vi "nanocal -- nuclear schottky fit -- 2x2 -- V9.vi"() -> ()   [LabVIEW 2021] (continued)
 -> 2.000000000000   ,  \"θ\" -> 45.000000000000   ,  \"Reoff\" -> -2979591.836734697220   ,  \"Imoff\" -> 0.000000000000   ,  \"στ1\" -> 0.135403699680   ,  \"στS\" -> 0.000163058440   ,  \"στN\" -> 0.001967445367    |>   , \n\"IDS0550_220606_RAW_cal__ref_\" ->   <|    \"ζ\" -> 0.030650031864   ,  \"τ1\" -> 0.371061825507   ,  \"τS\" -> 0.019434774268   ,  \"τN\" -> 0.003191687976   ,  \"τC\" -> 0.001854354331   ,  \"κ0\" -> 0.000000005040   ,  \"mm1\" -> 0.000050590010   ,  \"mm2\" -> 0.021630629169   ,  \"mm3\" -> 0.374554924692   ,  \"T\" -> 0.820000000000   ,  \"B\" -> 2.000000000000   ,  \"θ\" -> 45.000000000000   ,  \"Reoff\" -> -1632653.061224489940   ,  \"Imoff\" -> 0.000000000000   ,  \"στ1\" -> 0.107047861270   ,  \"στS\" -> 0.000201030582   ,  \"στN\" -> 0.000503414357    |>   , \n\"IDS0550_220606_RAW_cal__sam_\" ->   <|    \"ζ\" -> 0.000000000000   ,  \"τ1\" -> 0.000000000000   ,  \"τS\" -> 0.000000000000   ,  \"τN\" -> 0.000000000000   ,  \"τC\" -> 0.000000000000   ,  \"κ0\" -> 0.000000000000   ,  \"mm1\" -> 0.000000000000   ,  \"mm2\" -> 0.000000000000   ,  \"mm3\" -> 0.000000000000   ,  \"T\" -> 0.820000000000   ,  \"B\" -> 2.000000000000   ,  \"θ\" -> 45.000000000000   ,  \"Reoff\" -> 0.000000000000   ,  \"Imoff\" -> 0.000000000000   ,  \"στ1\" -> 0.000000000000   ,  \"στS\" -> 0.000000000000   ,  \"στN\" -> 0.000000000000    |>   , \n\"IDS0551_220606_RAW_cal__ref_\" ->   <|    \"ζ\" -> 0.023490949621   ,  \"τ1\" -> 0.378878569703   ,  \"τS\" -> 0.026968462806   ,  \"τN\" -> 0.001819085143   ,  \"τC\" -> 0.002360831644   ,  \"κ0\" -> 0.000000007142   ,  \"mm1\" -> 0.000049999340   ,  \"mm2\" -> 0.029754158704   ,  \"mm3\" -> 0.380899038091   ,  \"T\" -> 1.120000000000   ,  \"B\" -> 2.000000000000   ,  \"θ\" -> 45.000000000000   ,  \"Reoff\" -> -959183.673469387924   ,  \"Imoff\" -> 0.000000000000   ,  \"στ1\" -> 0.190596529331   ,  \"στS\" -> 0.000292683710   ,  \"στN\" -> 0.000959345989    |>   , \n\"IDS0551_220606_RAW_cal__sam_\" ->   <|    \"ζ\" -> 0.000000000000   ,  \"τ1\" -> 0.000000000000   ,  \"τS\" -> 0.000000000000   ,  \"τN\" -> 0.000000000000   ,  \"τC\" -> 0.000000000000   ,  \"κ0\" -> 0.000000000000   ,  \"mm1\" -> 0.000000000000   ,  \"mm2\" -> 0.000000000000   ,  \"mm3\" -> 0.000000000000   ,  \"T\" -> 1.120000000000   ,  \"B\" -> 2.000000000000   ,  \"θ\" -> 45.000000000000   ,  \"Reoff\" -> 0.000000000000   ,  \"Imoff\" -> 0.000000000000   ,  \"στ1\" -> 0.000000000000   ,  \"στS\" -> 0.000000000000   ,  \"στN\" -> 0.000000000000    |>   , \n\"IDS0552_220606_RAW_cal__ref_\" ->   <|    \"ζ\" -> 0.016903896176   ,  \"τ1\" -> 0.389208085767   ,  \"τS\" -> 0.042839293805   ,  \"τN\" -> 0.001054381509   ,  \"τC\" -> 0.002700942117   ,  \"κ0\" -> 0.000000012752   ,  \"mm1\" -> 0.000042315056   ,  \"mm2\" -> 0.046078096141   ,  \"mm3\" -> 0.390424266131   ,  \"T\" -> 1.900000000000   ,  \"B\" -> 2.000000000000   ,  \"θ\" -> 45.000000000000   ,  \"Reoff\" -> -285714.285714285448   ,  \"Imoff\" -> 0.000000000000   ,  \"στ1\" -> 0.071680793743   ,  \"στS\" -> 0.000751471945   ,  \"στN\" -> 0.000020808748    |>   , \n\"IDS0552_220606_RAW_cal__sam_\" ->   <|    \"ζ\" -> 0.000000000000   ,  \"τ1\" -> 0.000000000000   ,  \"τS\" -> 0.000000000000   ,  \"τN\" -> 0.000000000000   ,  \"τC\" -> 0.000000000000   ,  \"κ0\" -> 0.000000000000   ,  \"mm1\" -> 0.000000000000   ,  \"mm2\" -> 0.000000000000   ,  \"mm3\" -> 0.000000000000   ,  \"T\" -> 1.900000000000   ,  \"B\" -> 2.000000000000   ,  \"θ\" -> 45.000000000000   ,  \"Reoff\" -> 0.000000000000   ,  \"Imoff\" -> 0.000000000000   ,  \"στ1\" -> 0.000000000000   ,  \"στS\" -> 0.000000000000   ,  \"στN\" -> 0.000000000000    |>   , \n\"IDS0553_220606_RAW_cal__ref_\" ->   <|    \"ζ\" -> 0.019034298387   ,  \"τ1\" -> 0.340685747660   ,  \"τS\" -> 0.012600728873   ,  \"τN\" -> 0.000836062096   ,  \"τC\" -> 0.002405907399   ,  \"κ0\" -> 0.000000015790   ,  \"mm1\" -> 0.000037942280   ,  \"mm2\" -> 0.015168856864   ,  \"mm3\" -> 0.341577406773   ,  \"T\" -> 2.300000000000   ,  \"B\" -> 2.000000000000   ,  \"θ\" -> 45.000000000000   ,  \"Reoff\" -> -346938.775510204024   ,  \"Imoff\" -> 0.000000000000   ,  \"στ1\" -> 0.043118413730   ,  \"στS\" -> 0.000142443187   ,  \"στN\" -> 0.000023036701    |>   , \n\"IDS0553_220606_RAW_cal__sam_\" ->   <|    \"ζ\" -> 0.000000000000   ,  \"τ1\" -> 0.000000000000   ,  \"τS\" -> 0.000000000000   ,  \"τN\" -> 0.000000000000   ,  \"τC\" -> 0.000000000000   ,  \"κ0\" -> 0.000000000000   ,  \"mm1\" -> 0.000000000000   ,  \"mm2\" -> 0.000000000000   ,  \"mm3\" -> 0.000000000000   ,  \"T\" -> 2.300000000000   ,  \"B\" -> 2.000000000000   ,  \"θ\" -> 45.000000000000   ,  \"Reoff\" -> 0.000000000000   ,  \"Imoff\" -> 0.000000000000   ,  \"στ1\" -> 0.000000000000   ,  \"στS\" -> 0.000000000000   ,  \"στN\" -> 0.000000000000    |>   , \n\"IDS0554_220606_RAW_cal__ref_\" ->   <|    \"ζ\" -> 0.019434711880   ,  \"τ1\" -> 0.338729084958   ,  \"τS\" -> 0.009688878082   ,  \"τN\" -> 0.000475618163   ,  \"τC\" -> 0.002360170204   ,  \"κ0\" -> 0.000000022449   ,  \"mm1\" -> 0.000036425186   ,  \"mm2\" -> 0.012182847072   ,  \"mm3\" -> 0.339232023205   ,  \"T\" -> 3.100000000000   ,  \"B\" -> 2.000000000000   ,  \"θ\" -> 45.000000000000   ,  \"Reoff\" -> -224489.795918367803   ,  \"Imoff\" -> 0.000000000000   ,  \"στ1\" -> 0.018790484107   ,  \"στS\" -> 0.000064367566   ,  \"στN\" -> 0.000007244630    |>   , \n\"IDS0554_220606_RAW_cal__sam_\" ->   <|    \"ζ\" -> 0.000000000000   ,  \"τ1\" -> 0.000000000000   ,  \"τS\" -> 0.000000000000   ,  \"τN\" -> 0.000000000000   ,  \"τC\" -> 0.000000000000   ,  \"κ0\" -> 0.000000000000   ,  \"mm1\" -> 0.000000000000   ,  \"mm2\" -> 0.000000000000   ,  \"mm3\" -> 0.000000000000   ,  \"T\" -> 3.100000000000   ,  \"B\" -> 2.000000000000   ,  \"θ\" -> 45.000000000000   ,  \"Reoff\" -> 0.000000000000   ,  \"Imoff\" -> 0.000000000000   ,  \"στ1\" -> 0.000000000000   ,  \"στS\" -> 0.000000000000   ,  \"στN\" -> 0.000000000000    |>   , \n\"IDS0555_220606_RAW_cal__ref_\" ->   <|    \"ζ\" -> 0.021952381066   ,  \"τ1\" -> 0.337915266866   ,  \"τS\" -> 0.005864517957   ,  \"τN\" -> 0.000285674383   ,  \"τC\" -> 0.001869482382   ,  \"κ0\" -> 0.000000055591   ,  \"mm1\" -> 0.000030729933   ,  \"mm2\" -> 0.007825098033   ,  \"mm3\" -> 0.338214124988   ,  \"T\" -> 5.700000000000   ,  \"B\" -> 2.000000000000   ,  \"θ\" -> 45.000000000000   ,  \"Reoff\" -> -102040.816326530650   ,  \"Imoff\" -> 0.000000000000   ,  \"στ1\" -> 0.018966360272   ,  \"στS\" -> 0.000034456720   ,  \"στN\" -> 0.000003385178    |>   , \n\"IDS0555_220606_RAW_cal__sam_\" ->   <|    \"ζ\" -> 0.000000000000   ,  \"τ1\" -> 0.000000000000   ,  \"τS\" -> 0.000000000000   ,  \"τN\" -> 0.000000000000   ,  \"τC\" -> 0.000000000000   ,  \"κ0\" -> 0.000000000000   ,  \"mm1\" -> 0.000000000000   ,  \"mm2\" -> 0.000000000000   ,  \"mm3\" -> 0.000000000000   ,  \"T\" -> 5.700000000000   ,  \"B\" -> 2.000000000000   ,  \"θ\" -> 45.000000000000   ,  \"Reoff\" -> 0.000000000000   ,  \"Imoff\" -> 0.000000000000   ,  \"στ1\" -> 0.000000000000   ,  \"στS\" -> 0.000000000000   ,  \"στN\" -> 0.000000000000    |>   , \n\"IDS0556_220606_RAW_cal__ref_\" ->   <|    \"ζ\" -> 0.018774663118   ,  \"τ1\" -> 0.223771999883   ,  \"τS\" -> 0.042172507139   ,  \"τN\" -> 0.000220913712   ,  \"τC\" -> 0.002321380026   ,  \"κ0\" -> 0.000000009770   ,  \"mm1\" -> 0.000040623453   ,  \"mm2\" -> 0.045188092517   ,  \"mm3\" -> 0.224054006985   ,  \"T\" -> 1.500000000000   ,  \"B\" -> 4.000000000000   ,  \"θ\" -> 45.000000000000   ,  \"Reoff\" -> -530612.244897959753   ,  \"Imoff\" -> 0.000000000000   ,  \"στ1\" -> 0.017095464532   ,  \"στS\" -> 0.000347466214   ,  \"στN\" -> 0.000004822339    |>   , \n\"IDS0556_220606_RAW_cal__sam_\" ->   <|    \"ζ\" -> 0.000000000000   ,  \"τ1\" -> 0.000000000000   ,  \"τS\" -> 0.000000000000   ,  \"τN\" -> 0.000000000000   ,  \"τC\" -> 0.000000000000   ,  \"κ0\" -> 0.000000000000   ,  \"mm1\" -> 0.000000000000   ,  \"mm2\" -> 0.000000000000   ,  \"mm3\" -> 0.000000000000   ,  \"T\" -> 1.500000000000   ,  \"B\" -> 4.000000000000   ,  \"θ\" -> 45.000000000000   ,  \"Reoff\" -> 0.000000000000   ,  \"Imoff\" -> 0.000000000000   ,  \"στ1\" -> 0.000000000000   ,  \"στS\" -> 0.000000000000   ,  \"στN\" -> 0.000000000000    |>   , \n\"IDS0559_220607_RAW_cal__ref_\" ->   <|    \"ζ\" -> 0.355714515528   ,  \"τ1\" -> 0.301914651842   ,  \"τS\" -> 0.015251938720   ,  \"τN\" -> 0.009436044938   ,  \"τC\" -> 0.000785444302   ,  \"κ0\" -> 0.000000000710   ,  \"mm1\" -> 0.000200413404   ,  \"mm2\" -> 0.020338541635   ,  \"mm3\" -> 0.315630998909   ,  \"T\" -> 0.170000000000   ,  \"B\" -> 2.000000000000   ,  \"θ\" -> 0.000000000000   ,  \"Reoff\" -> -74000000.000000000000   ,  \"Imoff\" -> 0.000000000000   ,  \"στ1\" -> 0.232297531792   ,  \"στS\" -> 0.000374376394   ,  \"στN\" -> 0.007678585568    |>   , \n\"IDS0559_220607_RAW_cal__sam_\" ->   <|    \"ζ\" -> 0.000000000000   ,  \"τ1\" -> 0.000000000000   ,  \"τS\" -> 0.000000000000   ,  \"τN\" -> 0.000000000000   ,  \"τC\" -> 0.000000000000   ,  \"κ0\" -> 0.000000000000   ,  \"mm1\" -> 0.000000000000   ,  \"mm2\" -> 0.000000000000   ,  \"mm3\" -> 0.000000000000   ,  \"T\" -> 0.170000000000   ,  \"B\" -> 2.000000000000   ,  \"θ\" -> 0.000000000000   ,  \"Reoff\" -> 0.000000000000   ,  \"Imoff\" -> 0.000000000000   ,  \"στ1\" -> 0.000000000000   ,  \"στS\" -> 0.000000000000   ,  \"στN\" -> 0.000000000000    |>   , \n\"IDS0560_220607_RAW_cal__ref_\" ->   <|    \"ζ\" -> 0.449635679893   ,  \"τ1\" -> 0.299060701269   ,  \"τS\" -> 0.016808041703   ,  \"τN\" -> 0.012305660826   ,  \"τC\" -> 0.000825775215   ,  \"κ0\" -> 0.000000000592   ,  \"mm1\" -> 0.000250217726   ,  \"mm2\" -> 0.023425417691   ,  \"mm3\" -> 0.318415103028   ,  \"T\" -> 0.150000000000   ,  \"B\" -> 2.000000000000   ,  \"θ\" -> 0.000000000000   ,  \"Reoff\" -> -98857142.857142850800   ,  \"Imoff\" -> 0.000000000000   ,  \"στ1\" -> 1.839545255469   ,  \"στS\" -> 0.000824368006   ,  \"στN\" -> 0.069201981467    |>   , \n\"IDS0560_220607_RAW_cal__sam_\" ->   <|    \"ζ\" -> 0.000000000000   ,  \"τ1\" -> 0.000000000000   ,  \"τS\" -> 0.000000000000   ,  \"τN\" -> 0.000000000000   ,  \"τC\" -> 0.000000000000   ,  \"κ0\" -> 0.000000000000   ,  \"mm1\" -> 0.000000000000   ,  \"mm2\" -> 0.000000000000   ,  \"mm3\" -> 0.000000000000   ,  \"T\" -> 0.150000000000   ,  \"B\" -> 2.000000000000   ,  \"θ\" -> 0.000000000000   ,  \"Reoff\" -> 0.000000000000   ,  \"Imoff\" -> 0.000000000000   ,  \"στ1\" -> 0.000000000000   ,  \"στS\" -> 0.000000000000   ,  \"στN\" -> 0.000000000000    |>   , \n\"IDS0561_220607_RAW_cal__ref_\" ->   <|    \"ζ\" -> 0.668963686378   ,  \"τ1\" -> 0.239112055774   ,  \"τS\" -> 0.021396471169   ,  \"τN\" -> 0.016347037663   ,  \"τC\" -> 0.000866848111   ,  \"κ0\" -> 0.000000000434   ,  \"mm1\" -> 0.000342420854   ,  \"mm2\" -> 0.032017103471   ,  \"mm3\" -> 0.270611925197   ,  \"T\" -> 0.120000000000   ,  \"B\" -> 2.000000000000   ,  \"θ\" -> 0.000000000000   ,  \"Reoff\" -> -192285714.285714298000   ,  \"Imoff\" -> 0.000000000000   ,  \"στ1\" -> 1.100347031208   ,  \"στS\" -> 0.002027710728   ,  \"στN\" -> 0.065388411976    |>   , \n\"IDS0561_220607_RAW_cal__sam_\" ->   <|    \"ζ\" -> 0.000000000000   ,  \"τ1\" -> 0.000000000000   ,  \"τS\" -> 0.000000000000   ,  \"τN\" -> 0.000000000000   ,  \"τC\" -> 0.000000000000   ,  \"κ0\" -> 0.000000000000   ,  \"mm1\" -> 0.000000000000   ,  \"mm2\" -> 0.000000000000   ,  \"mm3\" -> 0.000000000000   ,  \"T\" -> 0.120000000000   ,  \"B\" -> 2.000000000000   ,  \"θ\" -> 0.000000000000   ,  \"Reoff\" -> 0.000000000000   ,  \"Imoff\" -> 0.000000000000   ,  \"στ1\" -> 0.000000000000   ,  \"στS\" -> 0.000000000000   ,  \"στN\" -> 0.000000000000    |>   , \n\"IDS0562_220607_RAW_cal__ref_\" ->   <|    \"ζ\" -> 0.258991387788   ,  \"τ1\" -> 0.317151511252   ,  \"τS\" -> 0.013390047800   ,  \"τN\" -> 0.006328285333   ,  \"τC\" -> 0.000848770466   ,  \"κ0\" -> 0.000000000905   ,  \"mm1\" -> 0.000167822844   ,  \"mm2\" -> 0.017085435691   ,  \"mm3\" -> 0.325572234779   ,  \"T\" -> 0.200000000000   ,  \"B\" -> 2.000000000000   ,  \"θ\" -> 0.000000000000   ,  \"Reoff\" -> -44857142.857142865700   ,  \"Imoff\" -> 0.000000000000   ,  \"στ1\" -> 0.531664595642   ,  \"στS\" -> 0.000229891647   ,  \"στN\" -> 0.006046488522    |>   , \n\"IDS0562_220607_RAW_cal__sam_\" ->   <|    \"ζ\" -> 0.000000000000   ,  \"τ1\" -> 0.000000000000   ,  \"τS\" -> 0.000000000000   ,  \"τN\" -> 0.000000000000   ,  \"τC\" -> 0.000000000000   ,  \"κ0\" -> 0.000000000000   ,  \"mm1\" -> 0.000000000000   ,  \"mm2\" -> 0.000000000000   ,  \"mm3\" -> 0.000000000000   ,  \"T\" -> 0.200000000000   ,  \"B\" -> 2.000000000000   ,  \"θ\" -> 0.000000000000   ,  \"Reoff\" -> 0.000000000000   ,  \"Imoff\" -> 0.000000000000   ,  \"στ1\" -> 0.000000000000   ,  \"στS\" -> 0.000000000000   ,  \"στN\" -> 0.000000000000    |>   , \n\"IDS0563_220607_RAW_cal__ref_\" ->   <|    \"ζ\" -> 0.172150656876   ,  \"τ1\" -> 0.349830224606   ,  \"τS\" -> 0.011998498670   ,  \"τN\" -> 0.004489980914   ,  \"τC\" -> 0.000896743670   ,  \"κ0\" -> 0.000000001200   ,  \"mm1\" -> 0.000124849196   ,  \"mm2\" -> 0.014606727837   ,  \"mm3\" -> 0.355322373419   ,  \"T\" -> 0.250000000000   ,  \"B\" -> 2.000000000000   ,  \"θ\" -> 0.000000000000   ,  \"Reoff\" -> -26000000.000000000000   ,  \"Imoff\" -> 0.000000000000   ,  \"στ1\" -> 0.049625629402   ,  \"στS\" -> 0.000087536047   ,  \"στN\" -> 0.000631838919    |>   , \n\"IDS0563_220607_RAW_cal__sam_\" ->   <|    \"ζ\" -> 0.000000000000   ,  \"τ1\" -> 0.000000000000   ,  \"τS\" -> 0.000000000000   ,  \"τN\" -> 0.000000000000   ,  \"τC\" -> 0.000000000000   ,  \"κ0\" -> 0.000000000000   ,  \"mm1\" -> 0.000000000000   ,  \"mm2\" -> 0.000000000000   ,  \"mm3\" -> 0.000000000000   ,  \"T\" -> 0.250000000000   ,  \"B\" -> 2.000000000000   ,  \"θ\" -> 0.000000000000   ,  \"Reoff\" -> 0.000000000000   ,  \"Imoff\" -> 0.000000000000   ,  \"στ1\" -> 0.000000000000   ,  \"στS\" -> 0.000000000000   ,  \"στN\" -> 0.000000000000    |>   , \n\"IDS0564_220607_RAW_cal__ref_\" ->   <|    \"ζ\" -> 0.118516574313   ,  \"τ1\" -> 0.350390004709   ,  \"τS\" -> 0.011220444254   ,  \"τN\" -> 0.003404891640   ,  \"τC\" -> 0.001143718862   ,  \"κ0\" -> 0.000000001568   ,  \"mm1\" -> 0.000111980338   ,  \"mm2\" -> 0.013430301860   ,  \"mm3\" -> 0.354350121975   ,  \"T\" -> 0.300000000000   ,  \"B\" -> 2.000000000000   ,  \"θ\" -> 0.000000000000   ,  \"Reoff\" -> -11428571.428571432800   ,  \"Imoff\" -> 0.000000000000   ,  \"στ1\" -> 0.301334297831   ,  \"στS\" -> 0.000157213626   ,  \"στN\" -> 0.004248705404    |>   , \n\"IDS0564_220607_RAW_cal__sam_\" ->   <|    \"ζ\" -> 0.000000000000   ,  \"τ1\" -> 0.000000000000   ,  \"τS\" -> 0.000000000000   ,  \"τN\" -> 0.000000000000   ,  \"τC\" -> 0.000000000000   ,  \"κ0\" -> 0.000000000000   ,  \"mm1\" -> 0.000000000000   ,  \"mm2\" -> 0.000000000000   ,  \"mm3\" -> 0.000000000000   ,  \"T\" -> 0.300000000000   ,  \"B\" -> 2.000000000000   ,  \"θ\" -> 0.000000000000   ,  \"Reoff\" -> 0.000000000000   ,  \"Imoff\" -> 0.000000000000   ,  \"στ1\" -> 0.000000000000   ,  \"στS\" -> 0.000000000000   ,  \"στN\" -> 0.000000000000    |>   , \n\"IDS0565_220607_RAW_cal__ref_\" ->   <|    \"ζ\" -> 0.087986482080   ,  \"τ1\" -> 0.256186322762   ,  \"τS\" -> 0.011079357499   ,  \"τN\" -> 0.003568927376   ,  \"τC\" -> 0.001270661793   ,  \"κ0\" -> 0.000000001939   ,  \"mm1\" -> 0.000093617177   ,  \"mm2\" -> 0.013023417519   ,  \"mm3\" -> 0.260277085788   ,  \"T\" -> 0.360000000000   ,  \"B\" -> 2.000000000000   ,  \"θ\" -> 0.000000000000   ,  \"Reoff\" -> -8000000.000000000000   ,  \"Imoff\" -> 0.000000000000   ,  \"στ1\" -> 0.066076122842   ,  \"στS\" -> 0.000113449498   ,  \"στN\" -> 0.000256105794    |>   , \n\"IDS0565_220607_RAW_cal__sam_\" ->   <|    \"ζ\" -> 0.000000000000   ,  \"τ1\" -> 0.000000000000   ,  \"τS\" -> 0.000000000000   ,  \"τN\" -> 0.000000000000   ,  \"τC\" -> 0.000000000000   ,  \"κ0\" -> 0.000000000000   ,  \"mm1\" -> 0.000000000000   ,  \"mm2\" -> 0.000000000000   ,  \"mm3\" -> 0.000000000000   ,  \"T\" -> 0.360000000000   ,  \"B\" -> 2.000000000000   ,  \"θ\" -> 0.000000000000   ,  \"Reoff\" -> 0.000000000000   ,  \"Imoff\" -> 0.000000000000   ,  \"στ1\" -> 0.000000000000   ,  \"στS\" -> 0.000000000000   ,  \"στN\" -> 0.000000000000    |>   , \n\"IDS0566_220607_RAW_cal__ref_\" ->   <|    \"ζ\" -> 0.070156403527   ,  \"τ1\" -> 0.262147223577   ,  \"τS\" -> 0.011262923295   ,  \"τN\" -> 0.002364637934   ,  \"τC\" -> 0.001329677258   ,  \"κ0\" -> 0.000000002344   ,  \"mm1\" -> 0.000078974457   ,  \"mm2\" -> 0.013170019334   ,  \"mm3\" -> 0.264811528958   ,  \"T\" -> 0.420000000000   ,  \"B\" -> 2.000000000000   ,  \"θ\" -> 0.000000000000   ,  \"Reoff\" -> -6285714.285714268690   ,  \"Imoff\" -> 0.000000000000   ,  \"στ1\" -> 0.014203019449   ,  \"στS\" -> 0.000120077801   ,  \"στN\" -> 0.000048266431    |>   , \n\"IDS0566_220607_RAW_cal__sam_\" ->   <|    \"ζ\" -> 0.000000000000   ,  \"τ1\" -> 0.000000000000   ,  \"τS\" -> 0.000000000000   ,  \"τN\" -> 0.000000000000   ,  \"τC\" -> 0.000000000000   ,  \"κ0\" -> 0.000000000000   ,  \"mm1\" -> 0.000000000000   ,  \"mm2\" -> 0.000000000000   ,  \"mm3\" -> 0.000000000000   ,  \"T\" -> 0.420000000000   ,  \"B\" -> 2.000000000000   ,  \"θ\" -> 0.000000000000   ,  \"Reoff\" -> 0.000000000000   ,  \"Imoff\" -> 0.000000000000   ,  \"στ1\" -> 0.000000000000   ,  \"στS\" -> 0.000000000000   ,  \"στN\" -> 0.000000000000    |>   , \n\"IDS0567_220607_RAW_cal__ref_\" ->   <|    \"ζ\" -> 0.052694231594   ,  \"τ1\" -> 0.206237698748   ,  \"τS\" -> 0.012180702952   ,  \"τN\" -> 0.001670150721   ,  \"τC\" -> 0.001358485752   ,  \"κ0\" -> 0.000000003021   ,  \"mm1\" -> 0.000061755571   ,  \"mm2\" -> 0.013991387047   ,  \"mm3\" -> 0.208123755646   ,  \"T\" -> 0.520000000000   ,  \"B\" -> 2.000000000000   ,  \"θ\" -> 0.000000000000   ,  \"Reoff\" -> -4571428.571428567170   ,  \"Imoff\" -> 0.000000000000   ,  \"στ1\" -> 0.013542176029   ,  \"στS\" -> 0.000128345810   ,  \"στN\" -> 0.000027133680    |>   , \n\"IDS0567_220607_RAW_cal__sam_\" ->   <|    \"ζ\" -> 0.000000000000   ,  \"τ1\" -> 0.000000000000   ,  \"τS\" -> 0.000000000000   ,  \"τN\" -> 0.000000000000   ,  \"τC\" -> 0.000000000000   ,  \"κ0\" -> 0.000000000000   ,  \"mm1\" -> 0.000000000000   ,  \"mm2\" -> 0.000000000000   ,  \"mm3\" -> 0.000000000000   ,  \"T\" -> 0.520000000000   ,  \"B\" -> 2.000000000000   ,  \"θ\" -> 0.000000000000   ,  \"Reoff\" -> 0.000000000000   ,  \"Imoff\" -> 0.000000000000   ,  \"στ1\" -> 0.000000000000   ,  \"στS\" -> 0.000000000000   ,  \"στN\" -> 0.000000000000    |>   , \n\"IDS0568_220607_RAW_cal__ref_\" ->   <|    \"ζ\" -> 0.042136652692   ,  \"τ1\" -> 0.203636345776   ,  \"τS\" -> 0.013404195797   ,  \"τN\" -> 0.001074940238   ,  \"τC\" -> 0.001728340244   ,  \"κ0\" -> 0.000000003726   ,  \"mm1\" -> 0.000062435783   ,  \"mm2\" -> 0.015542386487   ,  \"mm3\" -> 0.204849102111   ,  \"T\" -> 0.620000000000   ,  \"B\" -> 2.000000000000   ,  \"θ\" -> 0.000000000000   ,  \"Reoff\" -> -2612244.897959183900   ,  \"Imoff\" -> 0.000000000000   ,  \"στ1\" -> 0.011688220611   ,  \"στS\" -> 0.000121966623   ,  \"στN\" -> 0.000019089189    |>   , \n\"IDS0568_220607_RAW_cal__sam_\" ->   <|    \"ζ\" -> 0.000000000000   ,  \"τ1\" -> 0.000000000000   ,  \"τS\" -> 0.000000000000   ,  \"τN\" -> 0.000000000000   ,  \"τC\" -> 0.000000000000   ,  \"κ0\" -> 0.000000000000   ,  \"mm1\" -> 0.000000000000   ,  \"mm2\" -> 0.000000000000   ,  \"mm3\" -> 0.000000000000   ,  \"T\" -> 0.620000000000   ,  \"B\" -> 2.000000000000   ,  \"θ\" -> 0.000000000000   ,  \"Reoff\" -> 0.000000000000   ,  \"Imoff\" -> 0.000000000000   ,  \"στ1\" -> 0.000000000000   ,  \"στS\" -> 0.000000000000   ,  \"στN\" -> 0.000000000000    |>   , \n\"IDS0569_220607_RAW_cal__ref_\" ->   <|    \"ζ\" -> 0.030235387858   ,  \"τ1\" -> 0.200849812033   ,  \"τS\" -> 0.016889405709   ,  \"τN\" -> 0.000765333865   ,  \"τC\" -> 0.002360193521   ,  \"κ0\" -> 0.000000005110   ,  \"mm1\" -> 0.000061183035   ,  \"mm2\" -> 0.019613778642   ,  \"mm3\" -> 0.201723581349   ,  \"T\" -> 0.820000000000   ,  \"B\" -> 2.000000000000   ,  \"θ\" -> 0.000000000000   ,  \"Reoff\" -> -1142857.142857141790   ,  \"Imoff\" -> 0.000000000000   ,  \"στ1\" -> 0.016798355334   ,  \"στS\" -> 0.000164505064   ,  \"στN\" -> 0.000022903136    |>   , \n\"IDS0569_220607_RAW_cal__sam_\" ->   <|    \"ζ\" -> 0.000000000000   ,  \"τ1\" -> 0.000000000000   ,  \"τS\" -> 0.000000000000   ,  \"τN\" -> 0.000000000000   ,  \"τC\" -> 0.000000000000   ,  \"κ0\" -> 0.000000000000   ,  \"mm1\" -> 0.000000000000   ,  \"mm2\" -> 0.000000000000   ,  \"mm3\" -> 0.000000000000   ,  \"T\" -> 0.820000000000   ,  \"B\" -> 2.000000000000   ,  \"θ\" -> 0.000000000000   ,  \"Reoff\" -> 0.000000000000   ,  \"Imoff\" -> 0.000000000000   ,  \"στ1\" -> 0.000000000000   ,  \"στS\" -> 0.000000000000   ,  \"στN\" -> 0.000000000000    |>   , \n\"IDS0570_220607_RAW_cal__ref_\" ->   <|    \"ζ\" -> 0.023186603119   ,  \"τ1\" -> 0.069304039551   ,  \"τS\" -> 0.024728755203   ,  \"τN\" -> 0.000615822915   ,  \"τC\" -> 0.002362965503   ,  \"κ0\" -> 0.000000007147   ,  \"mm1\" -> 0.000049060818   ,  \"mm2\" -> 0.027208827859   ,  \"mm3\" -> 0.070341349169   ,  \"T\" -> 1.120000000000   ,  \"B\" -> 2.000000000000   ,  \"θ\" -> 0.000000000000   ,  \"Reoff\" -> -897959.183673471211   ,  \"Imoff\" -> 0.000000000000   ,  \"στ1\" -> 0.007066895477   ,  \"στS\" -> 0.000207495874   ,  \"στN\" -> 0.000024034388    |>   , \n\"IDS0570_220607_RAW_cal__sam_\" ->   <|    \"ζ\" -> 0.000000000000   ,  \"τ1\" -> 0.000000000000   ,  \"τS\" -> 0.000000000000   ,  \"τN\" -> 0.000000000000   ,  \"τC\" -> 0.000000000000   ,  \"κ0\" -> 0.000000000000   ,  \"mm1\" -> 0.000000000000   ,  \"mm2\" -> 0.000000000000   ,  \"mm3\" -> 0.000000000000   ,  \"T\" -> 1.120000000000   ,  \"B\" -> 2.000000000000   ,  \"θ\" -> 0.000000000000   ,  \"Reoff\" -> 0.000000000000   ,  \"Imoff\" -> 0.000000000000   ,  \"στ1\" -> 0.000000000000   ,  \"στS\" -> 0.000000000000   ,  \"στN\" -> 0.000000000000    |>   , \n\"IDS0571_220607_RAW_cal__ref_\" ->   <|    \"ζ\" -> 0.015770363513   ,  \"τ1\" -> 0.071971798635   ,  \"τS\" -> 0.047933574846   ,  \"τN\" -> 0.000365152941   ,  \"τC\" -> 0.002700044906   ,  \"κ0\" -> 0.000000012652   ,  \"mm1\" -> 0.000039747850   ,  \"mm2\" -> 0.050478715429   ,  \"mm3\" -> 0.073213796543   ,  \"T\" -> 1.900000000000   ,  \"B\" -> 2.000000000000   ,  \"θ\" -> 0.000000000000   ,  \"Reoff\" -> -285714.285714287310   ,  \"Imoff\" -> 0.000000000000   ,  \"στ1\" -> 0.006975803229   ,  \"στS\" -> 0.000442024056   ,  \"στN\" -> 0.000016462134    |>   , \n\"IDS0571_220607_RAW_cal__sam_\" ->   <|    \"ζ\" -> 0.000000000000   ,  \"τ1\" -> 0.000000000000   ,  \"τS\" -> 0.000000000000   ,  \"τN\" -> 0.000000000000   ,  \"τC\" -> 0.000000000000   ,  \"κ0\" -> 0.000000000000   ,  \"mm1\" -> 0.000000000000   ,  \"mm2\" -> 0.000000000000   ,  \"mm3\" -> 0.000000000000   ,  \"T\" -> 1.900000000000   ,  \"B\" -> 2.000000000000   ,  \"θ\" -> 0.000000000000   ,  \"Reoff\" -> 0.000000000000   ,  \"Imoff\" -> 0.000000000000   ,  \"στ1\" -> 0.000000000000   ,  \"στS\" -> 0.000000000000   ,  \"στN\" -> 0.000000000000    |>   , \n\"IDS0572_220607_RAW_cal__ref_\" ->   <|    \"ζ\" -> 0.018018584104   ,  \"τ1\" -> 0.047661155544   ,  \"τS\" -> 0.013484677326   ,  \"τN\" -> 0.000256030731   ,  \"τC\" -> 0.002573709531   ,  \"κ0\" -> 0.000000016044   ,  \"mm1\" -> 0.000038452225   ,  \"mm2\" -> 0.016129638273   ,  \"mm3\" -> 0.048055070739   ,  \"T\" -> 2.300000000000   ,  \"B\" -> 2.000000000000   ,  \"θ\" -> 0.000000000000   ,  \"Reoff\" -> -285714.285714287310   ,  \"Imoff\" -> 0.000000000000   ,  \"στ1\" -> 0.009039480993   ,  \"στS\" -> 0.000292801167   ,  \"στN\" -> 0.000013350378    |>   , \n\"IDS0572_220607_RAW_cal__sam_\" ->   <|    \"ζ\" -> 0.000000000000   ,  \"τ1\" -> 0.000000000000   ,  \"τS\" -> 0.000000000000   ,  \"τN\" -> 0.000000000000   ,  \"τC\" -> 0.000000000000   ,  \"κ0\" -> 0.000000000000   ,  \"mm1\" -> 0.000000000000   ,  \"mm2\" -> 0.000000000000   ,  \"mm3\" -> 0.000000000000   ,  \"T\" -> 2.300000000000   ,  \"B\" -> 2.000000000000   ,  \"θ\" -> 0.000000000000   ,  \"Reoff\" -> 0.000000000000   ,  \"Imoff\" -> 0.000000000000   ,  \"στ1\" -> 0.000000000000   ,  \"στS\" -> 0.000000000000   ,  \"στN\" -> 0.000000000000    |>   , \n\"IDS0573_220607_RAW_cal__ref_\" ->   <|    \"ζ\" -> 0.017854709230   ,  \"τ1\" -> 0.048990500372   ,  \"τS\" -> 0.009409191095   ,  \"τN\" -> 0.000133052666   ,  \"τC\" -> 0.002613702785   ,  \"κ0\" -> 0.000000022548   ,  \"mm1\" -> 0.000036125485   ,  \"mm2\" -> 0.012110331944   ,  \"mm3\" -> 0.049170363477   ,  \"T\" -> 3.100000000000   ,  \"B\" -> 2.000000000000   ,  \"θ\" -> 0.000000000000   ,  \"Reoff\" -> -163265.306122448295   ,  \"Imoff\" -> 0.000000000000   ,  \"στ1\" -> 0.003929388168   ,  \"στS\" -> 0.000082158552   ,  \"στN\" -> 0.000004662808    |>   , \n\"IDS0573_220607_RAW_cal__sam_\" ->   <|    \"ζ\" -> 0.000000000000   ,  \"τ1\" -> 0.000000000000   ,  \"τS\" -> 0.000000000000   ,  \"τN\" -> 0.000000000000   ,  \"τC\" -> 0.000000000000   ,  \"κ0\" -> 0.000000000000   ,  \"mm1\" -> 0.000000000000   ,  \"mm2\" -> 0.000000000000   ,  \"mm3\" -> 0.000000000000   ,  \"T\" -> 3.100000000000   ,  \"B\" -> 2.000000000000   ,  \"θ\" -> 0.000000000000   ,  \"Reoff\" -> 0.000000000000   ,  \"Imoff\" -> 0.000000000000   ,  \"στ1\" -> 0.000000000000   ,  \"στS\" -> 0.000000000000   ,  \"στN\" -> 0.000000000000    |>   , \n\"IDS0574_220607_RAW_cal__ref_\" ->   <|    \"ζ\" -> 0.021296069589   ,  \"τ1\" -> 0.048193111718   ,  \"τS\" -> 0.005769221839   ,  \"τN\" -> 0.000085869671   ,  \"τC\" -> 0.001966024103   ,  \"κ0\" -> 0.000000055540   ,  \"mm1\" -> 0.000030859965   ,  \"mm2\" -> 0.007810308294   ,  \"mm3\" -> 0.048297749508   ,  \"T\" -> 5.700000000000   ,  \"B\" -> 2.000000000000   ,  \"θ\" -> 0.000000000000   ,  \"Reoff\" -> -89795.918367346749   ,  \"Imoff\" -> 0.000000000000   ,  \"στ1\" -> 0.003900504752   ,  \"στS\" -> 0.000042384921   ,  \"στN\" -> 0.000002866550    |>   , \n\"IDS0574_220607_RAW_cal__sam_\" ->   <|    \"ζ\" -> 0.000000000000   ,  \"τ1\" -> 0.000000000000   ,  \"τS\" -> 0.000000000000   ,  \"τN\" -> 0.000000000000   ,  \"τC\" -> 0.000000000000   ,  \"κ0\" -> 0.000000000000   ,  \"mm1\" -> 0.000000000000   ,  \"mm2\" -> 0.000000000000   ,  \"mm3\" -> 0.000000000000   ,  \"T\" -> 5.700000000000   ,  \"B\" -> 2.000000000000   ,  \"θ\" -> 0.000000000000   ,  \"Reoff\" -> 0.000000000000   ,  \"Imoff\" -> 0.000000000000   ,  \"στ1\" -> 0.000000000000   ,  \"στS\" -> 0.000000000000   ,  \"στN\" -> 0.000000000000    |>   , \n\"IDS0578_220608_RAW_cal__ref_\" ->   <|    \"ζ\" -> 0.260580240331   ,  \"τ1\" -> 0.233392220968   ,  \"τS\" -> 0.019337528339   ,  \"τN\" -> 0.006746984129   ,  \"τC\" -> 0.000809912718   ,  \"κ0\" -> 0.000000000898   ,  \"mm1\" -> 0.000163092082   ,  \"mm2\" -> 0.024046559857   ,  \"mm3\" -> 0.242874102744   ,  \"T\" -> 0.200000000000   ,  \"B\" -> 2.000000000000   ,  \"θ\" -> 90.000000000000   ,  \"Reoff\" -> -51020408.163265287900   ,  \"Imoff\" -> 0.000000000000   ,  \"στ1\" -> 0.360874017703   ,  \"στS\" -> 0.000459944418   ,  \"στN\" -> 0.007141056200    |>   , \n\"IDS0578_220608_RAW_cal__sam_\" ->   <|    \"ζ\" -> 0.000000000000   ,  \"τ1\" -> 0.000000000000   ,  \"τS\" -> 0.000000000000   ,  \"τN\" -> 0.000000000000   ,  \"τC\" -> 0.000000000000   ,  \"κ0\" -> 0.000000000000   ,  \"mm1\" -> 0.000000000000   ,  \"mm2\" -> 0.000000000000   ,  \"mm3\" -> 0.000000000000   ,  \"T\" -> 0.200000000000   ,  \"B\" -> 2.000000000000   ,  \"θ\" -> 90.000000000000   ,  \"Reoff\" -> 0.000000000000   ,  \"Imoff\" -> 0.000000000000   ,  \"στ1\" -> 0.000000000000   ,  \"στS\" -> 0.000000000000   ,  \"στN\" -> 0.000000000000    |>   , \n\"IDS0579_220608_RAW_cal__ref_\" ->   <|    \"ζ\" -> 0.358041732305   ,  \"τ1\" -> 0.218984893341   ,  \"τS\" -> 0.022109893709   ,  \"τN\" -> 0.011578421119   ,  \"τC\" -> 0.000774433851   ,  \"κ0\" -> 0.000000000705   ,  \"mm1\" -> 0.000200343737   ,  \"mm2\" -> 0.028269791705   ,  \"mm3\" -> 0.237039329177   ,  \"T\" -> 0.170000000000   ,  \"B\" -> 2.000000000000   ,  \"θ\" -> 90.000000000000   ,  \"Reoff\" -> -83673469.387755096000   ,  \"Imoff\" -> 0.000000000000   ,  \"στ1\" -> 0.324633037067   ,  \"στS\" -> 0.000730773074   ,  \"στN\" -> 0.013143956795    |>   , \n\"IDS0579_220608_RAW_cal__sam_\" ->   <|    \"ζ\" -> 0.000000000000   ,  \"τ1\" -> 0.000000000000   ,  \"τS\" -> 0.000000000000   ,  \"τN\" -> 0.000000000000   ,  \"τC\" -> 0.000000000000   ,  \"κ0\" -> 0.000000000000   ,  \"mm1\" -> 0.000000000000   ,  \"mm2\" -> 0.000000000000   ,  \"mm3\" -> 0.000000000000   ,  \"T\" -> 0.170000000000   ,  \"B\" -> 2.000000000000   ,  \"θ\" -> 90.000000000000   ,  \"Reoff\" -> 0.000000000000   ,  \"Imoff\" -> 0.000000000000   ,  \"στ1\" -> 0.000000000000   ,  \"στS\" -> 0.000000000000   ,  \"στN\" -> 0.000000000000    |>   , \n\"IDS0580_220608_RAW_cal__ref_\" ->   <|    \"ζ\" -> 0.444194308226   ,  \"τ1\" -> 0.247703542844   ,  \"τS\" -> 0.025021615076   ,  \"τN\" -> 0.015371954390   ,  \"τC\" -> 0.000794757601   ,  \"κ0\" -> 0.000000000600   ,  \"mm1\" -> 0.000240752300   ,  \"mm2\" -> 0.033248610212   ,  \"mm3\" -> 0.273345101045   ,  \"T\" -> 0.150000000000   ,  \"B\" -> 2.000000000000   ,  \"θ\" -> 90.000000000000   ,  \"Reoff\" -> -104081632.653061211000   ,  \"Imoff\" -> 0.000000000000   ,  \"στ1\" -> 0.811876218659   ,  \"στS\" -> 0.001521304973   ,  \"στN\" -> 0.040822562310    |>   , \n\"IDS0580_220608_RAW_cal__sam_\" ->   <|    \"ζ\" -> 0.000000000000   ,  \"τ1\" -> 0.000000000000   ,  \"τS\" -> 0.000000000000   ,  \"τN\" -> 0.000000000000   ,  \"τC\" -> 0.000000000000   ,  \"κ0\" -> 0.000000000000   ,  \"mm1\" -> 0.000000000000   ,  \"mm2\" -> 0.000000000000   ,  \"mm3\" -> 0.000000000000   ,  \"T\" -> 0.150000000000   ,  \"B\" -> 2.000000000000   ,  \"θ\" -> 90.000000000000   ,  \"Reoff\" -> 0.000000000000   ,  \"Imoff\" -> 0.000000000000   ,  \"στ1\" -> 0.000000000000   ,  \"στS\" -> 0.000000000000   ,  \"στN\" -> 0.000000000000    |>   , \n\"IDS0581_220608_RAW_cal__ref_\" ->   <|    \"ζ\" -> 0.686806962981   ,  \"τ1\" -> 0.191964510357   ,  \"τS\" -> 0.031477597051   ,  \"τN\" -> 0.029789944795   ,  \"τC\" -> 0.000797477821   ,  \"κ0\" -> 0.000000000433   ,  \"mm1\" -> 0.000321816656   ,  \"mm2\" -> 0.040244297441   ,  \"mm3\" -> 0.255542390272   ,  \"T\" -> 0.120000000000   ,  \"B\" -> 2.000000000000   ,  \"θ\" -> 90.000000000000   ,  \"Reoff\" -> -218367346.938775510000   ,  \"Imoff\" -> 0.000000000000   ,  \"στ1\" -> 0.248597488998   ,  \"στS\" -> 0.002831181242   ,  \"στN\" -> 0.031806706752    |>   , \n\"IDS0581_220608_RAW_cal__sam_\" ->   <|    \"ζ\" -> 0.000000000000   ,  \"τ1\" -> 0.000000000000   ,  \"τS\" -> 0.000000000000   ,  \"τN\" -> 0.000000000000   ,  \"τC\" -> 0.000000000000   ,  \"κ0\" -> 0.000000000000   ,  \"mm1\" -> 0.000000000000   ,  \"mm2\" -> 0.000000000000   ,  \"mm3\" -> 0.000000000000   ,  \"T\" -> 0.120000000000   ,  \"B\" -> 2.000000000000   ,  \"θ\" -> 90.000000000000   ,  \"Reoff\" -> 0.000000000000   ,  \"Imoff\" -> 0.000000000000   ,  \"στ1\" -> 0.000000000000   ,  \"στS\" -> 0.000000000000   ,  \"στN\" -> 0.000000000000    |>   , \n\"IDS0582_220608_RAW_cal__ref_\" ->   <|    \"ζ\" -> 0.166369563634   ,  \"τ1\" -> 0.241506341921   ,  \"τS\" -> 0.016551953229   ,  \"τN\" -> 0.004476656392   ,  \"τC\" -> 0.000955255274   ,  \"κ0\" -> 0.000000001230   ,  \"mm1\" -> 0.000130674320   ,  \"mm2\" -> 0.019667491815   ,  \"mm3\" -> 0.247190561287   ,  \"T\" -> 0.250000000000   ,  \"B\" -> 2.000000000000   ,  \"θ\" -> 90.000000000000   ,  \"Reoff\" -> -23265306.122448980800   ,  \"Imoff\" -> 0.000000000000   ,  \"στ1\" -> 0.210252832674   ,  \"στS\" -> 0.000349343663   ,  \"στN\" -> 0.005793752107    |>   , \n\"IDS0582_220608_RAW_cal__sam_\" ->   <|    \"ζ\" -> 0.000000000000   ,  \"τ1\" -> 0.000000000000   ,  \"τS\" -> 0.000000000000   ,  \"τN\" -> 0.000000000000   ,  \"τC\" -> 0.000000000000   ,  \"κ0\" -> 0.000000000000   ,  \"mm1\" -> 0.000000000000   ,  \"mm2\" -> 0.000000000000   ,  \"mm3\" -> 0.000000000000   ,  \"T\" -> 0.250000000000   ,  \"B\" -> 2.000000000000   ,  \"θ\" -> 90.000000000000   ,  \"Reoff\" -> 0.000000000000   ,  \"Imoff\" -> 0.000000000000   ,  \"στ1\" -> 0.000000000000   ,  \"στS\" -> 0.000000000000   ,  \"στN\" -> 0.000000000000    |>   , \n\"IDS0583_220608_RAW_cal__ref_\" ->   <|    \"ζ\" -> 0.118361182005   ,  \"τ1\" -> 0.150636490656   ,  \"τS\" -> 0.015529851966   ,  \"τN\" -> 0.003531374182   ,  \"τC\" -> 0.001007690492   ,  \"κ0\" -> 0.000000001529   ,  \"mm1\" -> 0.000101358307   ,  \"mm2\" -> 0.017747047219   ,  \"mm3\" -> 0.155113111027   ,  \"T\" -> 0.300000000000   ,  \"B\" -> 2.000000000000   ,  \"θ\" -> 90.000000000000   ,  \"Reoff\" -> -15102040.816326528800   ,  \"Imoff\" -> 0.000000000000   ,  \"στ1\" -> 0.078929426255   ,  \"στS\" -> 0.000167827635   ,  \"στN\" -> 0.002346663512    |>   , \n\"IDS0583_220608_RAW_cal__sam_\" ->   <|    \"ζ\" -> 0.000000000000   ,  \"τ1\" -> 0.000000000000   ,  \"τS\" -> 0.000000000000   ,  \"τN\" -> 0.000000000000   ,  \"τC\" -> 0.000000000000   ,  \"κ0\" -> 0.000000000000   ,  \"mm1\" -> 0.000000000000   ,  \"mm2\" -> 0.000000000000   ,  \"mm3\" -> 0.000000000000   ,  \"T\" -> 0.300000000000   ,  \"B\" -> 2.000000000000   ,  \"θ\" -> 90.000000000000   ,  \"Reoff\" -> 0.000000000000   ,  \"Imoff\" -> 0.000000000000   ,  \"στ1\" -> 0.000000000000   ,  \"στS\" -> 0.000000000000   ,  \"στN\" -> 0.000000000000    |>   , \n\"IDS0584_220608_RAW_cal__ref_\" ->   <|    \"ζ\" -> 0.085716797729   ,  \"τ1\" -> 0.145541921942   ,  \"τS\" -> 0.014790459938   ,  \"τN\" -> 0.003022723579   ,  \"τC\" -> 0.001204929117   ,  \"κ0\" -> 0.000000001932   ,  \"mm1\" -> 0.000088946369   ,  \"mm2\" -> 0.016747642578   ,  \"mm3\" -> 0.149250334678   ,  \"T\" -> 0.360000000000   ,  \"B\" -> 2.000000000000   ,  \"θ\" -> 90.000000000000   ,  \"Reoff\" -> -8571428.571428582080   ,  \"Imoff\" -> 0.000000000000   ,  \"στ1\" -> 0.049017314235   ,  \"στS\" -> 0.000077215540   ,  \"στN\" -> 0.000273627633    |>   , \n\"IDS0584_220608_RAW_cal__sam_\" ->   <|    \"ζ\" -> 0.000000000000   ,  \"τ1\" -> 0.000000000000   ,  \"τS\" -> 0.000000000000   ,  \"τN\" -> 0.000000000000   ,  \"τC\" -> 0.000000000000   ,  \"κ0\" -> 0.000000000000   ,  \"mm1\" -> 0.000000000000   ,  \"mm2\" -> 0.000000000000   ,  \"mm3\" -> 0.000000000000   ,  \"T\" -> 0.360000000000   ,  \"B\" -> 2.000000000000   ,  \"θ\" -> 90.000000000000   ,  \"Reoff\" -> 0.000000000000   ,  \"Imoff\" -> 0.000000000000   ,  \"στ1\" -> 0.000000000000   ,  \"στS\" -> 0.000000000000   ,  \"στN\" -> 0.000000000000    |>   , \n\"IDS0585_220608_RAW_cal__ref_\" ->   <|    \"ζ\" -> 0.064153972834   ,  \"τ1\" -> 0.145990399088   ,  \"τS\" -> 0.014755700071   ,  \"τN\" -> 0.002470459255   ,  \"τC\" -> 0.001390626850   ,  \"κ0\" -> 0.000000002341   ,  \"mm1\" -> 0.000077364865   ,  \"mm2\" -> 0.016676693112   ,  \"mm3\" -> 0.148958253844   ,  \"T\" -> 0.420000000000   ,  \"B\" -> 2.000000000000   ,  \"θ\" -> 90.000000000000   ,  \"Reoff\" -> -4530612.244897958820   ,  \"Imoff\" -> 0.000000000000   ,  \"στ1\" -> 0.010117026609   ,  \"στS\" -> 0.000141538965   ,  \"στN\" -> 0.000077781764    |>   , \n\"IDS0585_220608_RAW_cal__sam_\" ->   <|    \"ζ\" -> 0.000000000000   ,  \"τ1\" -> 0.000000000000   ,  \"τS\" -> 0.000000000000   ,  \"τN\" -> 0.000000000000   ,  \"τC\" -> 0.000000000000   ,  \"κ0\" -> 0.000000000000   ,  \"mm1\" -> 0.000000000000   ,  \"mm2\" -> 0.000000000000   ,  \"mm3\" -> 0.000000000000   ,  \"T\" -> 0.420000000000   ,  \"B\" -> 2.000000000000   ,  \"θ\" -> 90.000000000000   ,  \"Reoff\" -> 0.000000000000   ,  \"Imoff\" -> 0.000000000000   ,  \"στ1\" -> 0.000000000000   ,  \"στS\" -> 0.000000000000   ,  \"στN\" -> 0.000000000000    |>   , \n\"IDS0586_220608_RAW_cal__ref_\" ->   <|    \"ζ\" -> 0.050400440296   ,  \"τ1\" -> 0.120007371635   ,  \"τS\" -> 0.015618683096   ,  \"τN\" -> 0.001956039129   ,  \"τC\" -> 0.001501517777   ,  \"κ0\" -> 0.000000002996   ,  \"mm1\" -> 0.000066249745   ,  \"mm2\" -> 0.017490709551   ,  \"mm3\" -> 0.122412426079   ,  \"T\" -> 0.520000000000   ,  \"B\" -> 2.000000000000   ,  \"θ\" -> 90.000000000000   ,  \"Reoff\" -> -3877551.020408162850   ,  \"Imoff\" -> 0.000000000000   ,  \"στ1\" -> 0.009823024060   ,  \"στS\" -> 0.000148546431   ,  \"στN\" -> 0.000049706708    |>   , \n\"IDS0586_220608_RAW_cal__sam_\" ->   <|    \"ζ\" -> 0.000000000000   ,  \"τ1\" -> 0.000000000000   ,  \"τS\" -> 0.000000000000   ,  \"τN\" -> 0.000000000000   ,  \"τC\" -> 0.000000000000   ,  \"κ0\" -> 0.000000000000   ,  \"mm1\" -> 0.000000000000   ,  \"mm2\" -> 0.000000000000   ,  \"mm3\" -> 0.000000000000   ,  \"T\" -> 0.520000000000   ,  \"B\" -> 2.000000000000   ,  \"θ\" -> 90.000000000000   ,  \"Reoff\" -> 0.000000000000   ,  \"Imoff\" -> 0.000000000000   ,  \"στ1\" -> 0.000000000000   ,  \"στS\" -> 0.000000000000   ,  \"στN\" -> 0.000000000000    |>   , \n\"IDS0587_220608_RAW_cal__ref_\" ->   <|    \"ζ\" -> 0.040966221247   ,  \"τ1\" -> 0.107264057054   ,  \"τS\" -> 0.017218763514   ,  \"τN\" -> 0.001743151532   ,  \"τC\" -> 0.001685988856   ,  \"κ0\" -> 0.000000003666   ,  \"mm1\" -> 0.000060834390   ,  \"mm2\" -> 0.019154933369   ,  \"mm3\" -> 0.109472991205   ,  \"T\" -> 0.620000000000   ,  \"B\" -> 2.000000000000   ,  \"θ\" -> 90.000000000000   ,  \"Reoff\" -> -2816326.530612244270   ,  \"Imoff\" -> 0.000000000000   ,  \"στ1\" -> 0.008843102756   ,  \"στS\" -> 0.000179440929   ,  \"στN\" -> 0.000073166949    |>   , \n\"IDS0587_220608_RAW_cal__sam_\" ->   <|    \"ζ\" -> 0.000000000000   ,  \"τ1\" -> 0.000000000000   ,  \"τS\" -> 0.000000000000   ,  \"τN\" -> 0.000000000000   ,  \"τC\" -> 0.000000000000   ,  \"κ0\" -> 0.000000000000   ,  \"mm1\" -> 0.000000000000   ,  \"mm2\" -> 0.000000000000   ,  \"mm3\" -> 0.000000000000   ,  \"T\" -> 0.620000000000   ,  \"B\" -> 2.000000000000   ,  \"θ\" -> 90.000000000000   ,  \"Reoff\" -> 0.000000000000   ,  \"Imoff\" -> 0.000000000000   ,  \"στ1\" -> 0.000000000000   ,  \"στS\" -> 0.000000000000   ,  \"στN\" -> 0.000000000000    |>   , \n\"IDS0588_220608_RAW_cal__ref_\" ->   <|    \"ζ\" -> 0.027966572573   ,  \"τ1\" -> 0.110878949003   ,  \"τS\" -> 0.020906801035   ,  \"τN\" -> 0.001317162593   ,  \"τC\" -> 0.002396852626   ,  \"κ0\" -> 0.000000005050   ,  \"mm1\" -> 0.000058809998   ,  \"mm2\" -> 0.023466150465   ,  \"mm3\" -> 0.112596332885   ,  \"T\" -> 0.820000000000   ,  \"B\" -> 2.000000000000   ,  \"θ\" -> 90.000000000000   ,  \"Reoff\" -> -1020408.163265304640   ,  \"Imoff\" -> 0.000000000000   ,  \"στ1\" -> 0.009326447287   ,  \"στS\" -> 0.000184300760   ,  \"στN\" -> 0.000049241490    |>   , \n\"IDS0588_220608_RAW_cal__sam_\" ->   <|    \"ζ\" -> 0.000000000000   ,  \"τ1\" -> 0.000000000000   ,  \"τS\" -> 0.000000000000   ,  \"τN\" -> 0.000000000000   ,  \"τC\" -> 0.000000000000   ,  \"κ0\" -> 0.000000000000   ,  \"mm1\" -> 0.000000000000   ,  \"mm2\" -> 0.000000000000   ,  \"mm3\" -> 0.000000000000   ,  \"T\" -> 0.820000000000   ,  \"B\" -> 2.000000000000   ,  \"θ\" -> 90.000000000000   ,  \"Reoff\" -> 0.000000000000   ,  \"Imoff\" -> 0.000000000000   ,  \"στ1\" -> 0.000000000000   ,  \"στS\" -> 0.000000000000   ,  \"στN\" -> 0.000000000000    |>   , \n\"IDS0589_220608_RAW_cal__ref_\" ->   <|    \"ζ\" -> 0.023281533249   ,  \"τ1\" -> 0.113795019123   ,  \"τS\" -> 0.028800719763   ,  \"τN\" -> 0.000699230708   ,  \"τC\" -> 0.002435159498   ,  \"κ0\" -> 0.000000007137   ,  \"mm1\" -> 0.000051258085   ,  \"mm2\" -> 0.031580340212   ,  \"mm3\" -> 0.114785334873   ,  \"T\" -> 1.120000000000   ,  \"B\" -> 2.000000000000   ,  \"θ\" -> 90.000000000000   ,  \"Reoff\" -> -938775.510204080491   ,  \"Imoff\" -> 0.000000000000   ,  \"στ1\" -> 0.007362854909   ,  \"στS\" -> 0.000278698493   ,  \"στN\" -> 0.000011047668    |>   , \n\"IDS0589_220608_RAW_cal__sam_\" ->   <|    \"ζ\" -> 0.000000000000   ,  \"τ1\" -> 0.000000000000   ,  \"τS\" -> 0.000000000000   ,  \"τN\" -> 0.000000000000   ,  \"τC\" -> 0.000000000000   ,  \"κ0\" -> 0.000000000000   ,  \"mm
